vi "Example Output.vi"() -> ()   [LabVIEW 2013]
uses:
  C:/tf/play/labview/Tinkerforge.dll
  Tinkerforge.dll
panel:
  in  "uid":string="xyz"
  in  "port":i32=4223
  in  "host":string="localhost"
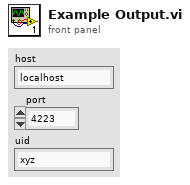
[diagram p1: front panel]
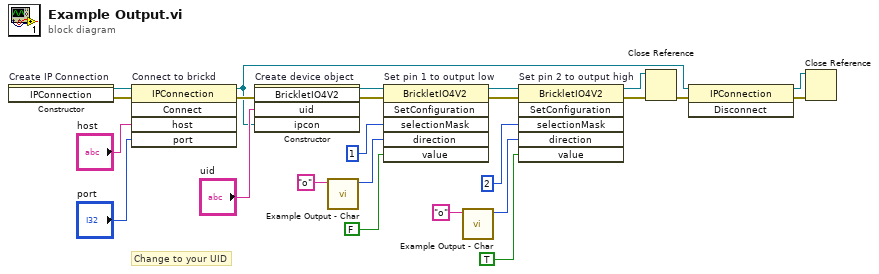
[diagram p0: block diagram]
diagram:
  # "Change to your UID"
  n1 = constructor on="Create IP Connection" class="IPConnection"() -> (reference out=w24:refnum<k24>, error out=w13:errorcluster)  [unwired: 3 in, 1 out]
  n2 = invoke on="Connect to brickd" class="IPConnection" method="Connect"(reference=w24, error in=w13, "host"="host", "port"="port") -> (reference out=w15:refnum<k24>, error out=w20:errorcluster)  [unwired: 1 in, 3 out]
  n3 = constructor on="Create device object" class="BrickletIO4V2"(error in=w20, "uid"="uid", "ipcon"=w15) -> (reference out=w18:refnum<k24>, error out=w19:errorcluster)  [unwired: 2 in, 3 out]
  n4 = call "Example Output - Char.vi"("string"="o") -> ("char"=w6:u16)  [unwired: 10 in]
  n5 = invoke on="Set pin 1 to output low" class="BrickletIO4V2" method="SetConfiguration"(reference=w18, error in=w19, "selectionMask"=u8 1 ("channel"), "direction"=w6, "value"=FALSE) -> (reference out=w10:refnum<k24>, error out=w11:errorcluster)  [unwired: 1 in, 4 out]
  n6 = call "Example Output - Char.vi"("string"="o") -> ("char"=w4:u16)  [unwired: 10 in]
  n7 = invoke on="Set pin 2 to output high" class="BrickletIO4V2" method="SetConfiguration"(reference=w10, error in=w11, "selectionMask"=u8 2 ("channel"), "direction"=w4, "value"=TRUE) -> (reference out=w9:refnum<k24>, error out=w8:errorcluster)  [unwired: 1 in, 4 out]
  n8 = Close Reference(reference=w9, error in (no error)=w8) -> (error out=w17:errorcluster)
  n9 = invoke class="IPConnection" method="Disconnect"(reference=w15, error in=w17) -> (reference out=w14:refnum<k24>, error out=w16:errorcluster)  [unwired: 1 in, 1 out]
  n10 = Close Reference(reference=w14, error in (no error)=w16) -> ()  [unwired: 1 out]
